vi "labeling_2_sub.vi"(11 "Refnum in":refnum<k33>) -> (2 "TEH WANTED POINT":dbl format="%#_13g", 3 "Array":T1(array[cluster]))   [LabVIEW 2020]
uses:
  Global Variables/Global_Rating.vi
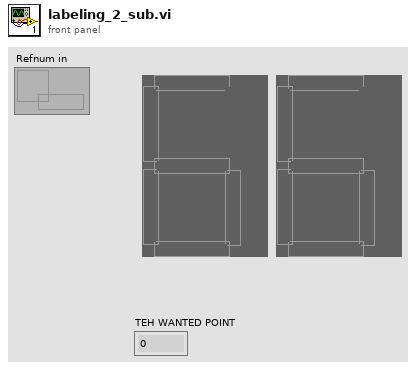
[diagram p1: front panel]
types:
  T1 = cluster{"Boolean":bool, "Boolean 2":bool, "Boolean 3":bool, "Boolean 4":bool, "Boolean 5":bool, "Boolean 6":bool, "Boolean 7":bool}[]
  T2 = cluster{"t[0]":bool, "t[1]":bool, "t[2]":bool, "t[3]":bool, "t[4]":bool, "t[5]":bool, "t[6]":bool}
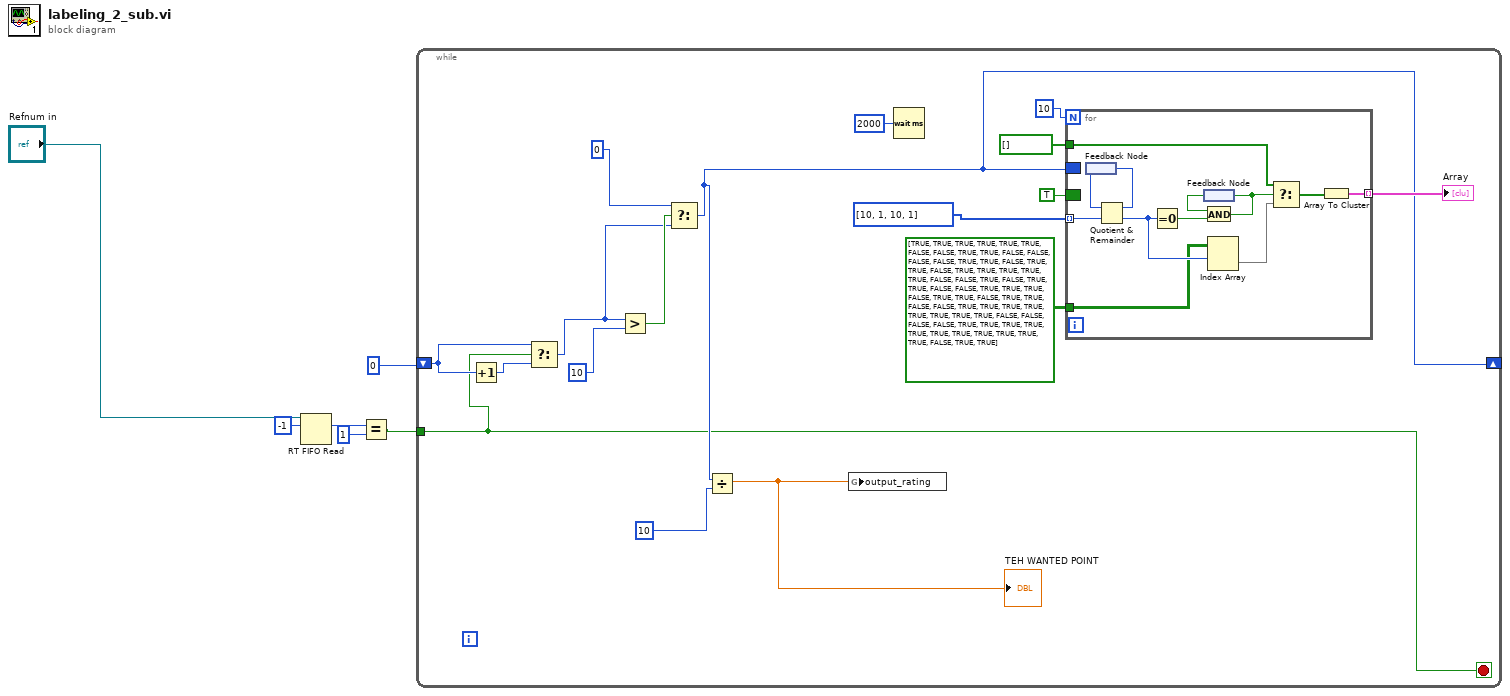
[diagram p0: block diagram]
diagram:
  n1 = RT FIFO Read(0:"Refnum in", 1:i8 -1 ("element")) -> (9:w2:i16)  [unwired: 2 in, 4 out]
  n2 = Equal?(x=w2, y=i8 1) -> (x = y?=w5:bool)
  n3 = while {
    shift-right: [w12] -> _
    shift-left: 0 -> [w11]
    tunnel: w5 -> [w7]
    stop <- w7 stop-if-true
    n4 = Increment(x=w11) -> (x+1=w10:i32)
    n5 = Select(t=w11, s=w7, f=w10) -> (s? t:f=w9:i32)
    n6 = Greater?(x=w9, y=10) -> (0:w13:bool)
    n7 = Select(t=0, s=w13, f=w9) -> (s? t:f=w12:i32)
    n8 = Divide(x=w12, y=10) -> (x/y=w16:dbl)
    "TEH WANTED POINT" <- w16
    n9 = global write "Global_Rating.vi" "output_rating"(w16) -> ()
    n10 = Wait (ms)(milliseconds to wait=u32 2000) -> ()  [unwired: 1 out]
    n11 = for {
      N: 10 -> [_]
      border: w12 -> [_]
      tunnel: i32[] [10, 1, 10, 1] -> [w33] mode=indexing
      tunnel: [w32] -> w23 mode=indexing
      border: TRUE -> [_]
      tunnel: bool[][] [[TRUE, TRUE, TRUE, TRUE, TRUE, TRUE, FALSE], [FALSE, TRUE, TRUE, FALSE, FALSE, FALSE, FALSE], [TRUE, TRUE, FALSE, TRUE, TRUE, FALSE, TRUE], [TRUE, TRUE, TRUE, TRUE, FALSE, FALSE, TRUE], [FALSE, TRUE, TRUE, FALSE, FALSE, TRUE, TRUE], [TRUE, FALSE, TRUE, TRUE, FALSE, TRUE, TRUE], [FALSE, FALSE, TRUE, TRUE, TRUE, TRUE, TRUE], [TRUE, TRUE, TRUE, FALSE, FALSE, FALSE, FALSE], [TRUE, TRUE, TRUE, TRUE, TRUE, TRUE, TRUE], [TRUE, TRUE, TRUE, TRUE, FALSE, TRUE, TRUE]] -> [w25]
      tunnel: bool[] [] ("t") -> [w24]
      n12 = feedback #1() -> (w34:i32)
      n13 = Quotient & Remainder(x=w34, y=w33) -> (x-y*floor(x/y)=w35:i32, floor(x/y)=w31:i32)
      n14 = feedback-in #1(w35) -> ()
      n15 = Equal To 0?(x=w31) -> (x = 0?=w30:bool)
      n16 = feedback #2() -> (w29:bool)
      n17 = And(x=w29, y=w30) -> (x .and. y?=w26:bool)
      n18 = feedback-in #2(w26) -> ()
      n19 = Index Array(array=w25, index (row)=w31) -> (element=w28:bool[])  [unwired: 1 in]
      n20 = Select(t=w24, s=w26, f=w28) -> (s? t:f=w27:bool[])
      n21 = Array To Cluster(array=w27) -> (cluster=w32:T2)
    }
    "Array" <- w23
  }
